vi "B7_65_GPIB_Init.vi"(0 "DriverConnect in":T1={"InterfaceType"=enum."VISA", "OpenedSession"="", "InterfaceSettings"={"Interface"=enum."RS232", "EOS 4 read"=enum."LF (\\n)", "EOS 4 write"=enum."LF (\\n)", "TMO, ms"=10000, "Sett"=variant(cluster{"Baud Rate":u32, "Data Bits":u16, "Parity":u16, "Stop Bits":u16, "Flow Control":u16, "Eho":bool} {"Baud Rate"=75, "Data Bits"=0, "Parity"=0, "Stop Bits"=0, "Flow Control"=0, "Eho"=FALSE})}}, 11 "error in":T8, 13 "Driver Name":T7="B1_28", 14 "Error Code":T6=5490) -> (4 "DriverConnect out":T1={"InterfaceType"=enum."VISA", "OpenedSession"="", "InterfaceSettings"={"Interface"=enum."RS232", "EOS 4 read"=enum."LF (\\n)", "EOS 4 write"=enum."LF (\\n)", "TMO, ms"=10000, "Sett"=variant(cluster{"Baud Rate":u32, "Data Bits":u16, "Parity":u16, "Stop Bits":u16, "Flow Control":u16, "Eho":bool} {"Baud Rate"=75, "Data Bits"=0, "Parity"=0, "Stop Bits"=0, "Flow Control"=0, "Eho"=FALSE})}}, 8 "Not Found response":bool, 15 "error out":T8)   [LabVIEW 2018]
uses:
  MOKO_LabViewLibrary/MokoLowLevel/MokoLowLovelControl/MLLC_Error.ctl
  MOKO_LabViewLibrary/MokoLowLevel/MokoLowLovelControl/MLLC_DriverName.ctl
  MOKO_LabViewLibrary/MokoLowLevel/MokoLowLovelControl/MLLC_ErrorCode.ctl
  MOKO_LabViewLibrary/MokoLowLevel/MokoLowLovelControl/MLLC_ConnectCluster.ctl
  MOKO_LabViewLibrary/MokoLowLevel/MokoLowLovelControl/MLLC_InterfaceType.ctl
  MOKO_LabViewLibrary/MokoLowLevel/MokoLowLovelControl/MLLC_OpenedSession.ctl
  MOKO_LabViewLibrary/MokoLowLevel/MokoLowLovelControl/MLLC_InterfaceSettings.ctl
  MOKO_LabViewLibrary/MokoLowLevel/MokoLowLovelControl/MLLC_InterfaceKind.ctl
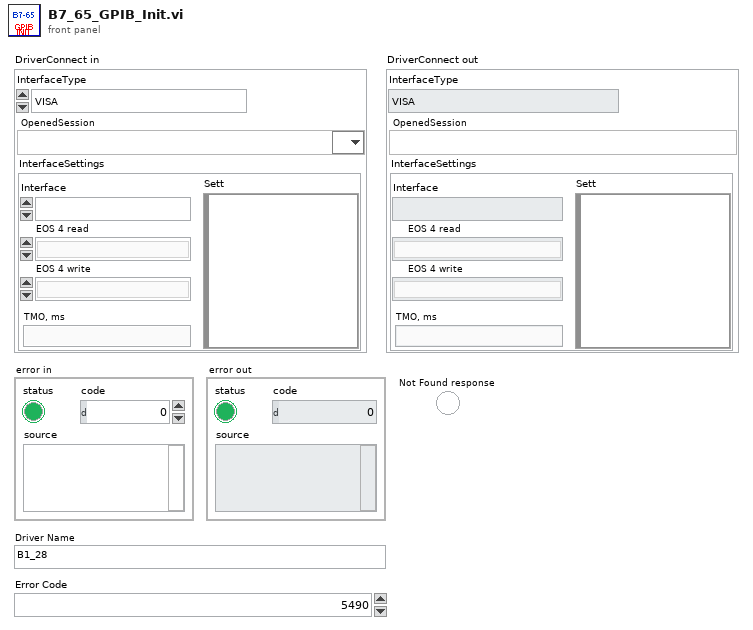
[diagram p1: front panel]
types:
  T1 = typedef "MLLC_ConnectCluster.ctl" = cluster{"InterfaceType":T2, "OpenedSession":T3, "InterfaceSettings":T4}
  T2 = typedef "MLLC_InterfaceType.ctl" = enum16{"VISA", "Prologix USB-GPIB"}
  T3 = typedef "MLLC_OpenedSession.ctl" = refnum<visa-resource-name>
  T4 = typedef "MLLC_InterfaceSettings.ctl" = cluster{"Interface":T5, "EOS 4 read":enum16{"Default (=EOS 4 write)", "CR (\\r)", "LF (\\n)", "None"}, "EOS 4 write":enum16{"CR+LF (\\r\\n)", "CR (\\r)", "LF (\\n)", "None"}, "TMO, ms":i32, "Sett":variant}
  T5 = typedef "MLLC_InterfaceKind.ctl" = enum16{"RS232", "GPIB", "USB", "Ethernet", "another"}
  T6 = typedef "MLLC_ErrorCode.ctl" = u32
  T7 = typedef "MLLC_DriverName.ctl" = string
  T8 = typedef "MLLC_Error.ctl" = errorcluster
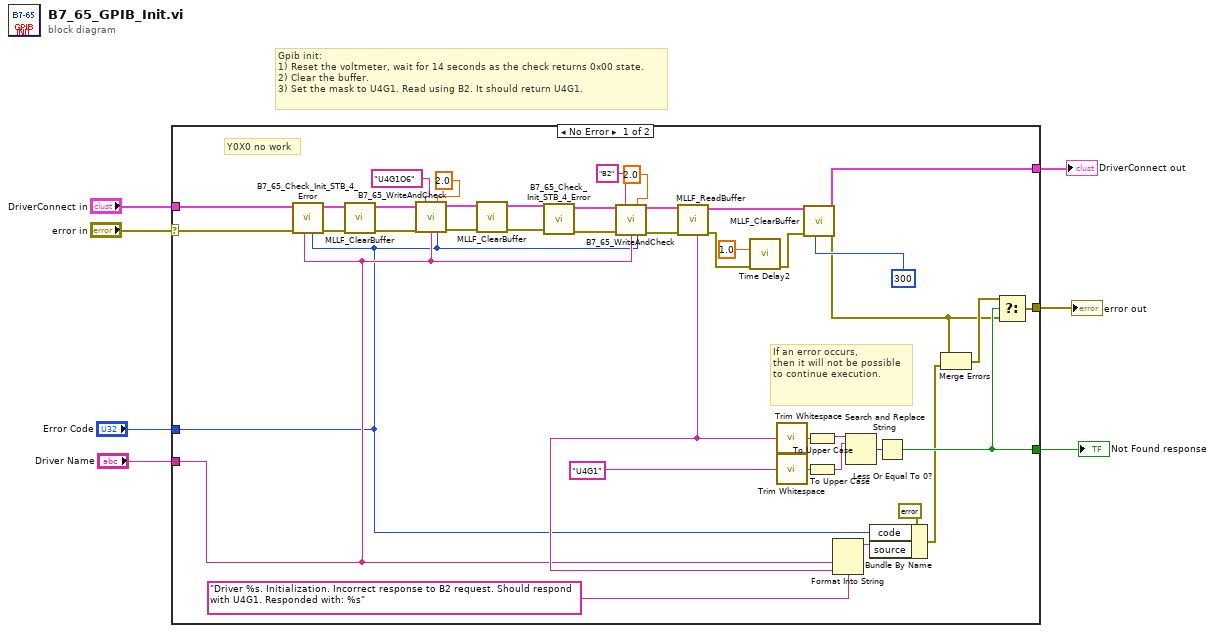
[diagram p0: block diagram]
diagram:
  # "Gpib init:\n1) Reset the voltmeter, wait for 14 seconds as the check returns 0x00 state.\n2) Clear the buffer.\n3) Set the mask to U4G1. Read using B2. It should return U4G1."
  n1 = case shown="No Error" "error in" {
    selector: "error in" -> [w32 w50]
    tunnel: [w40 w50] -> w7
    tunnel: [w34 w49] -> w1
    tunnel: "Error Code" -> [w10 _]
    tunnel: "Driver Name" -> [w11 _]
    tunnel: [w39 _] -> w3
    tunnel: "DriverConnect in" -> [w9 w49]
    frame No Error {
      # "If an error occurs,\nthen it will not be possible\nto continue execution."
      # "Y0X0 no work"
      n2 = call "B7_65_Check_Init_STB_4_Error.vi"("Error Code"=w10, "Driver Name"=w11, "error in"=w32, "DriverConnect in"=w9) -> ("error out"=w13:T8, "DriverConnect out"=w14:T1)  [unwired: 6 in]
      n3 = call "MLLF_ClearBuffer.vi"("Error In"=w13, "DriverConnect in"=w14) -> ("Error Out"=w27:errorcluster, "DriverConnect out"=w8:T1)  [unwired: 6 in, 1 out]
      n4 = call "B7_65_WriteAndCheck.vi"("DriverConnect in"=w8, "Str2Write"="U4G1O6" ("Request"), "Command Time (s)"=2.0, "error in"=w27, "Driver Name"=w11, "Error Code"=w10) -> ("DriverConnect out"=w25:T1, "error out"=w24:T8)  [unwired: 8 in]
      n5 = call "MLLF_ClearBuffer.vi"("Error In"=w24, "DriverConnect in"=w25) -> ("Error Out"=w22:errorcluster, "DriverConnect out"=w23:T1)  [unwired: 6 in, 1 out]
      n6 = call "B7_65_Check_Init_STB_4_Error.vi"("error in"=w22, "DriverConnect in"=w23) -> ("error out"=w16:T8, "DriverConnect out"=w17:T1)  [unwired: 8 in]
      n7 = call "B7_65_WriteAndCheck.vi"("DriverConnect in"=w17, "Str2Write"="B2" ("Request"), "Command Time (s)"=2.0, "error in"=w16, "Driver Name"=w11, "Error Code"=w10) -> ("DriverConnect out"=w19:T1, "error out"=w18:T8)  [unwired: 8 in]
      n8 = call "MLLF_ReadBuffer.vi"("Error In"=w18, "DriverConnect in"=w19) -> ("Error Out"=w15:errorcluster, "DriverConnect out"=w30:T1, "String"=w31:string)  [unwired: 6 in]
      n9 = call "Time Delay2"("error in (no error)"=w15, "Delay Time (s)"=1.0 ("Command Time (s)")) -> ("error out"=w29:errorcluster)  [unwired: 9 in]
      n10 = call <vilib>:"Trim Whitespace.vi"("string"=w31) -> ("trimmed string"=w48:string)  [unwired: 1 in]
      n11 = call <vilib>:"Trim Whitespace.vi"("string"="U4G1" ("Response")) -> ("trimmed string"=w47:string)  [unwired: 1 in]
      n12 = call "MLLF_ClearBuffer.vi"("Timeout(default = 300 ms)"=u32 300 ("Timeout"), "Error In"=w29, "DriverConnect in"=w30) -> ("Error Out"=w33:errorcluster, "DriverConnect out"=w34:T1)  [unwired: 5 in, 1 out]
      n13 = To Upper Case(1:w48) -> (0:w46:string)
      n14 = To Upper Case(1:w47) -> (0:w45:string)
      n15 = Format Into String(format string="Driver %s. Initialization. Incorrect response to B2 request. Should respond with U4G1. Responded with: %s", w11, w31) -> (resulting string=w42:string)  [unwired: 2 in, 1 out]
      n16 = Search and Replace String(input string=w46, search string=w45) -> (number of replacements=w44:i32)  [unwired: 6 in, 3 out]
      n17 = Bundle By Name(cluster=errorcluster {"status"=TRUE, "code"=0, "source"=""} ("error in"), "code"=w10, "source"=w42) -> (w37:errorcluster)
      n18 = Less Or Equal To 0?(x=w44) -> (x <= 0?=w39:bool)
      n19 = Merge Errors(w33, w37) -> (w36:errorcluster)
      n20 = Select(t=w36, s=w39, f=w33) -> (s? t:f=w40:errorcluster)
    }
    frame Error {
    }
  }
  "error out" <- w7
  "Not Found response" <- w3
  "DriverConnect out" <- w1
